vi "CleanUp.vi"(8 "error in (no error)":errorcluster, 11 "Prueba10 in":refnum<class "Prueba10.lvclass">) -> (0 "error out":errorcluster, 3 "Prueba10 out":refnum<class "Prueba10.lvclass">)   [LabVIEW 2019, in "Prueba10.lvclass"]
uses:
  Prueba10.lvclass
  C:/Users/ivan_/Documents/procal/Pruebas/Prueba/Prueba.lvclass
  Prueba/Prueba.lvclass/Prueba.ctl
  Prueba10.lvclass/Prueba10.ctl
  Base de Datos/SQLiteConnector/SQLiteConnection.lvclass
  Base de Datos/Base de Datos.lvclass
  Prueba/Prueba.lvclass
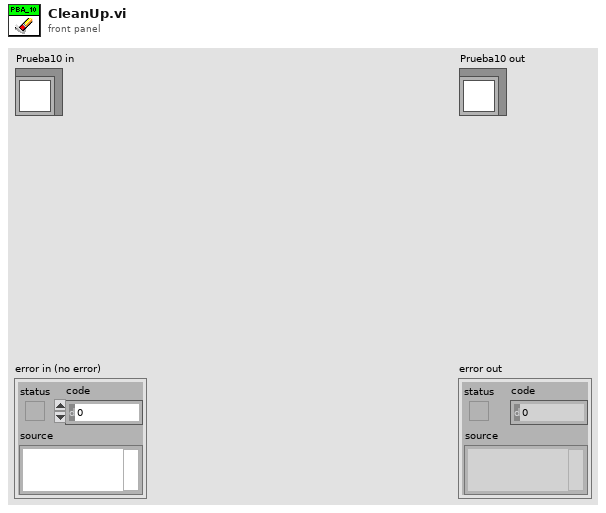
[diagram p1: front panel]
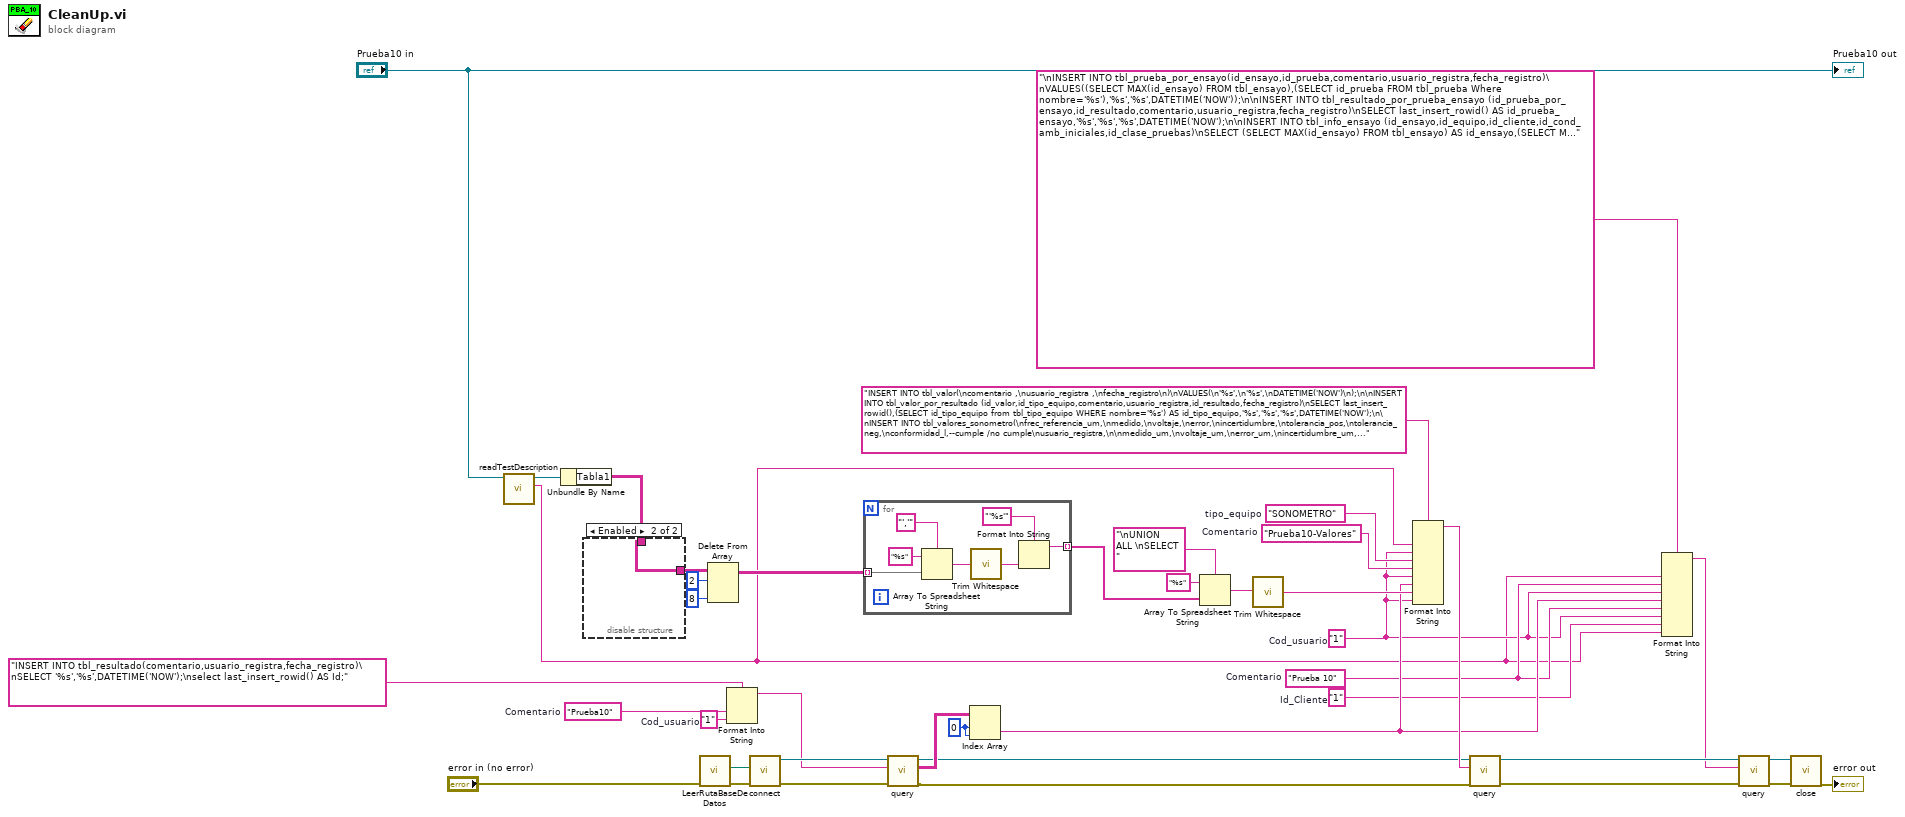
[diagram p0: block diagram]
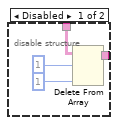
[diagram p2: hidden frame]
diagram:
  w14 = "1"  # Id_Cliente
  w15 = "Prueba 10"  # Comentario
  w24 = "SONOMETRO"  # tipo_equipo
  w23 = "Prueba10-Valores"  # Comentario
  w29 = 0 ("index (row)")
  w31 = "1"  # Cod_usuario
  w32 = "Prueba10"  # Comentario
  w13 = "1"  # Cod_usuario
  n1 = call "readTestDescription.vi"("Prueba in"="Prueba10 in") -> ("Test Description"=w5:string, "Prueba out"=w6:refnum<class "Prueba10.lvclass">)  [unwired: 8 in, 1 out]
  n2 = Unbundle By Name(w6) -> ("Tabla1"=w8:string[][])
  n3 = disable-structure shown="Enabled" {
    disable-tunnel: [w44 w46] -> w10
    disable-tunnel: w8 -> [w43 w46]
    frame Disabled {
      n4 = Delete From Array(array=w43, length=1, index (col)=1 ("disabled index (col)")) -> (array with subset deleted=w44:string[][])  [unwired: 1 in, 1 out]
    }
    frame Enabled {
    }
  }
  n5 = call "LeerRutaBaseDeDatos.vi"("error in (no error)"="error in (no error)") -> ("error out"=w36:errorcluster, "Database Path"=w35:path)  [unwired: 9 in]
  n6 = Delete From Array(array=w10, length=2, index (col)=8 ("disabled index (col)")) -> (array with subset deleted=w11:string[][])  [unwired: 1 in, 1 out]
  n7 = Format Into String(format string="INSERT INTO tbl_resultado(comentario,usuario_registra,fecha_registro)\nSELECT '%s','%s',DATETIME('NOW');\nselect last_insert_rowid() AS Id;" ("SQL Statement"), w32, w31) -> (resulting string=w30:string)  [unwired: 2 in, 1 out]
  n8 = call "connect.vi"("error in (no error)"=w36, "Database Path"=w35) -> ("error out"=w28:errorcluster, "object out"=w33:refnum<class "SQLiteConnection.lvclass">)  [unwired: 8 in]
  n9 = for {
    tunnel: w11 -> [w47] mode=indexing
    tunnel: [w50] -> w39 mode=indexing
    n10 = Array To Spreadsheet String(delimiter (Tab)="','", array=w47, 3:"%s" ("format string")) -> (spreadsheet string=w49:string)
    n11 = call <vilib>:"Trim Whitespace.vi"("string"=w49) -> ("trimmed string"=w48:string)  [unwired: 1 in]
    n12 = Format Into String(format string="'%s'", w48) -> (resulting string=w50:string)  [unwired: 2 in, 1 out]
  }
  n13 = call "query.vi"("error in (no error)"=w28, "SQL Statement"=w30, "object in"=w33) -> ("error out"=w9:errorcluster, "result"=w27:string[][], "object out"=w26:refnum<class "SQLiteConnection.lvclass">)  [unwired: 5 in, 1 out]
  n14 = Index Array(array=w27, index (row)=w29, index (col)=w29) -> (element=w16:string)
  n15 = Array To Spreadsheet String(delimiter (Tab)="\nUNION ALL \nSELECT ", array=w39, 3:"%s" ("format string")) -> (spreadsheet string=w38:string)
  n16 = call <vilib>:"Trim Whitespace.vi"("string"=w38) -> ("trimmed string"=w25:string)  [unwired: 1 in]
  n17 = Format Into String(format string="INSERT INTO tbl_valor(\ncomentario ,\nusuario_registra ,\nfecha_registro\n)\nVALUES(\n'%s',\n'%s',\nDATETIME('NOW')\n);\n\nINSERT INTO tbl_valor_por_resultado (id_valor,id_tipo_equipo,comentario,usuario_registra,id_resultado,fecha_registro)\nSELECT last_insert_rowid(),(SELECT id_tipo_equipo from tbl_tipo_equipo WHERE nombre='%s') AS id_tipo_equipo,'%s','%s','%s',DATETIME('NOW');\n\nINSERT INTO tbl_valores_sonometro(\nfrec_referencia_um,\nmedido,\nvoltaje,\nerror,\nincertidumbre,\ntolerancia_pos,\ntolerancia_neg,\nconformidad_l,--cumple /no cumple\nusuario_registra,\n\nmedido_um,\nvoltaje_um,\nerror_um,\nincertidumbre_um,\ntolerancia_pos_um,\ntolerancia_neg_um,\n\nid_valor,\nfecha_registro\n)\nSELECT * FROM(\nSELECT %s\n) AS T\nINNER JOIN\n(SELECT %s AS usuario,'dB','mV','dB','dB','dB','dB',(SELECT MAX(id_valor) FROM tbl_valor) AS id_valor,DATETIME('NOW') fecha ) AS F;\n", w5, w13, w24, w23, w13, w16, w25, w13) -> (resulting string=w34:string)  [unwired: 2 in, 1 out]
  n18 = call "query.vi"("error in (no error)"=w9, "SQL Statement"=w34, "object in"=w26) -> ("error out"=w20:errorcluster, "object out"=w22:refnum<class "SQLiteConnection.lvclass">)  [unwired: 5 in, 2 out]
  n19 = Format Into String(format string="\nINSERT INTO tbl_prueba_por_ensayo(id_ensayo,id_prueba,comentario,usuario_registra,fecha_registro)\nVALUES((SELECT MAX(id_ensayo) FROM tbl_ensayo),(SELECT id_prueba FROM tbl_prueba Where nombre='%s'),'%s','%s',DATETIME('NOW'));\n\nINSERT INTO tbl_resultado_por_prueba_ensayo (id_prueba_por_ensayo,id_resultado,comentario,usuario_registra,fecha_registro)\nSELECT last_insert_rowid() AS id_prueba_ensayo,'%s','%s','%s',DATETIME('NOW');\n\nINSERT INTO tbl_info_ensayo (id_ensayo,id_equipo,id_cliente,id_cond_amb_iniciales,id_clase_pruebas)\nSELECT (SELECT MAX(id_ensayo) FROM tbl_ensayo) AS id_ensayo,(SELECT MAX(id_equipo) FROM tbl_equipo) AS id_equipo,'%s' AS id_cliente,(SELECT MAX(id_cond_amb_iniciales) FROM tbl_cond_amb_iniciales) AS id_cond_amb_iniciales,\n(SELECT id_clase_prueba FROM tbl_clase_prueba WHERE id_clase=(SELECT id_clase FROM tbl_equipo ORDER BY id_equipo DESC LIMIT 1)  AND id_prueba=(SELECT id_prueba FROM tbl_prueba Where nombre='%s')) AS id_clase_pruebas;\n", w5, w15, w13, w16, w15, w13, w14, w5) -> (resulting string=w17:string)  [unwired: 2 in, 1 out]
  n20 = call "query.vi"("error in (no error)"=w20, "SQL Statement"=w17, "object in"=w22) -> ("error out"=w19:errorcluster, "object out"=w21:refnum<class "SQLiteConnection.lvclass">)  [unwired: 5 in, 2 out]
  n21 = call-dynamic "close.vi"("error in (no error)"=w19, "object in"=w21) -> ("error out"=→"error out":errorcluster)  [unwired: 8 in, 1 out]
  "Prueba10 out" <- "Prueba10 in"
